vi "Set HSDIO Voltage Level for all Channels.vi"(8 "Low Level":dbl format="%.2p", 9 "High Level":dbl=1.8 format="%.2p", 10 "Pins":string[](array[string]), 11 "Semiconductor Module Context":T1) -> (0 "error out":errorcluster)   [LabVIEW 2013]
uses:
  <vilib>/NI_TestStand_SemiconductorModule/NI_TestStand_Semiconductor_Module.lvlibp/PinMap/General/SemiconductorModuleContext.ctl
  <vilib>/NI_TestStand_SemiconductorModule/NI_TestStand_Semiconductor_Module.lvlibp/PinMap/HSDIO/PinsToNIHSDIOSessions.vi
  <instrlib>/niHSDIO/niHSDIO.llb/niHSDIO Configure Data Voltage Custom Levels.vi
  <vilib>/NI_TestStand_SemiconductorModule/NI_TestStand_Semiconductor_Module.lvlibp
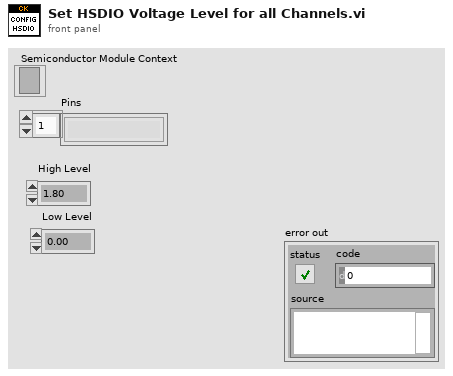
[diagram p1: front panel]
types:
  T1 = typedef "NI_TestStand_Semiconductor_Module.lvlibp/SemiconductorModuleContext.ctl" = refnum<k7>
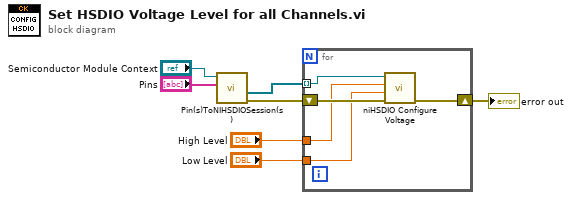
[diagram p0: block diagram]
diagram:
  n1 = call-poly <vilib>:"Pin(s)ToNIHSDIOSession(s).vi"("Pins"="Pins", "Semiconductor Module Context"="Semiconductor Module Context") -> ("error out"=w7:errorcluster, "Generation Sessions"=w6:refnum<k15>[])  [unwired: 4 in, 4 out]
  n2 = for {
    shift-right: [w8] -> w4
    shift-left: w7 -> [w12]
    tunnel: w6 -> [w11] mode=indexing
    tunnel: "High Level" -> [w10]
    tunnel: "Low Level" -> [w9]
    n3 = call-poly <instrlib>:"niHSDIO Configure Voltage.vi"("error in (no error)"=w12, "low level (0.00 volts)"=w9, "high level (3.30 volts)"=w10, "instrument handle"=w11) -> ("error out"=w8:errorcluster)  [unwired: 6 in, 1 out]
  }
  "error out" <- w4
